vi "Create Pattern Script - Cmd Frame.vi"(8 "error in (no error)":errorcluster, 11 "BML Pattern Creater in":refnum<class "BML Pattern Creater.lvclass">) -> (0 "error out":errorcluster, 2 "CMD Frame out":string, 3 "BML Pattern Creater out":refnum<class "BML Pattern Creater.lvclass">)   [LabVIEW 2018, in "BML Pattern Creater.lvlib" / "BML Pattern Creater.lvclass"]
uses:
  BML Pattern Creater.lvclass
  Special Frame.ctl
  BML Pattern Creater.lvclass/BML Pattern Creater.ctl
  Interfaces/Protocol Interface.lvlibp/Interfaces/Protocol Interface/Pin State.ctl
  Read Frame Data.vi
  Interfaces/Protocol Interface.lvlibp/Interfaces/Protocol Interface/Protocol Interface.lvclass
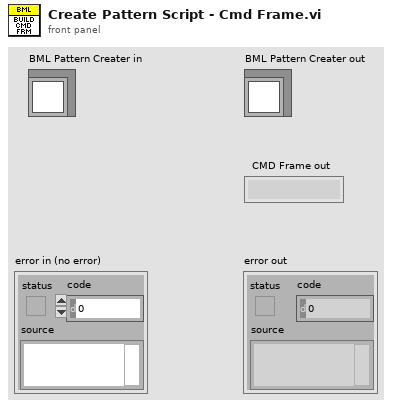
[diagram p1: front panel]
types:
  T1 = typedef "BML Pattern Creater.lvlib/BML Pattern Creater.lvclass/Special Frame.ctl" = enum16{"Sync Header", "BML Header", "SW Trig", "SetID State", "Exit SetID State", "SW Reset", "Wait"}
  T2 = typedef "FRM Data - BML.ctl" = cluster{"Pattern_Name":string, "Data":u8[], "Start_Addr":u16, "ChipID":u8, "num of wait ms":i8, "Opcode":string[], "BML OM":T3, "BurstLength":T4, "FSN":u8, "R/W?":T5}
  T3 = typedef "OM - BML.ctl" = enum16{"Normal", "ImmeEffect", "InitSlaveID", "LoadData"}
  T4 = typedef "Burst Length.ctl" = enum8{"0", "2", "3", "4", "5", "8", "16", "32"}
  T5 = typedef "RW Options.ctl" = enum16{"Read", "Write", "R/W"}
  T6 = typedef "Protocol Interface.lvlibp/Protocol Interface.lvclass/Pin State.ctl" = enum16{"0", "1", "L", "H", "X", "V", "D", "M"}
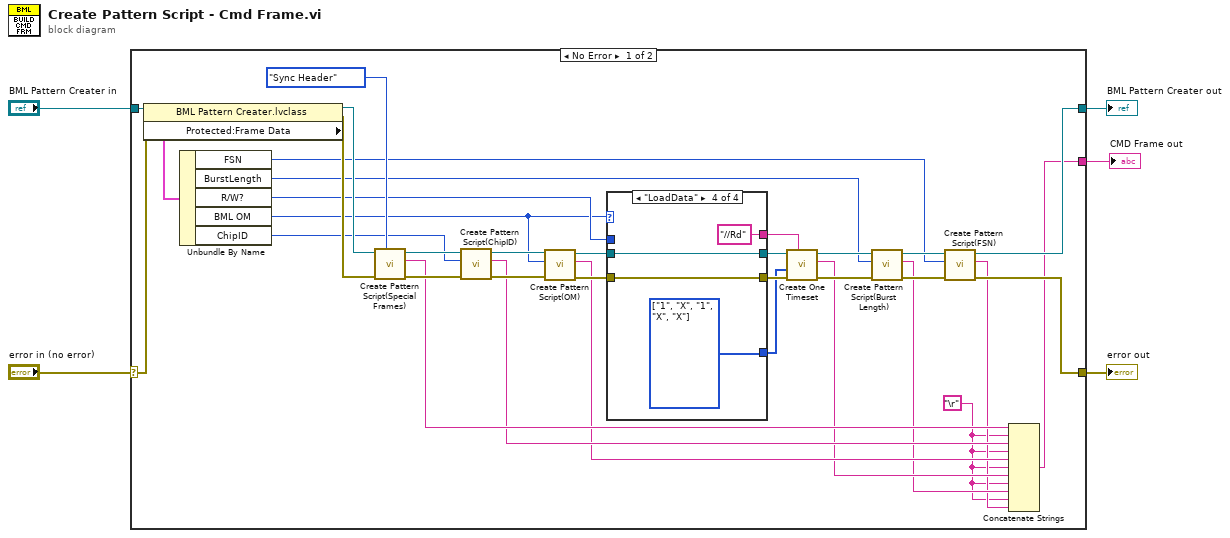
[diagram p0: block diagram]
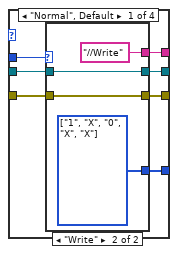
[diagram p2: hidden frame]
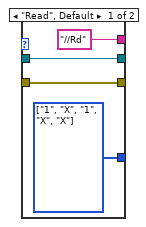
[diagram p3: hidden frame]
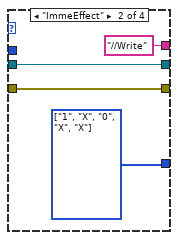
[diagram p4: hidden frame]
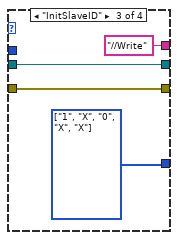
[diagram p5: hidden frame]
diagram:
  n1 = case shown="No Error" "error in (no error)" {
    selector: "error in (no error)" -> [w39 w69]
    tunnel: [w14 w69] -> w4
    tunnel: [w15 w68] -> w2
    tunnel: "BML Pattern Creater in" -> [w40 w68]
    tunnel: [w6 _] -> w1
    frame No Error {
      w7 = "\r"
      n2 = property class="BML Pattern Creater.lvclass"(reference=w40, error in=w39) -> (reference out=w37:refnum<class "BML Pattern Creater.lvclass">, error out=w36:errorcluster, "Protected:Frame Data"=w38:T2)
      n3 = Unbundle By Name(w38) -> ("FSN"=w16:u8, "BurstLength"=w17:T4, "R/W?"=w27:T5, "BML OM"=w19:T3, "ChipID"=w32:u8)
      n4 = call "Create Pattern Script(Special Frames).vi"("Special Frame Type"=Special_Frame."Sync Header", "error in (no error)"=w36, "BML Pattern Creater in"=w37) -> ("error out"=w33:errorcluster, "string out"=w13:string, "BML Pattern Creater out"=w34:refnum<class "BML Pattern Creater.lvclass">)  [unwired: 6 in]
      n5 = call "Create Pattern Script(ChipID).vi"("error in (no error)"=w33, "ChipID"=w32, "BML Pattern Creater in"=w34) -> ("error out"=w31:errorcluster, "Script out"=w12:string, "BML Pattern Creater out"=w30:refnum<class "BML Pattern Creater.lvclass">)  [unwired: 6 in]
      n6 = call "Create Pattern Script(OM).vi"("error in (no error)"=w31, "BML OM"=w19, "BML Pattern Creater in"=w30) -> ("error out"=w26:errorcluster, "OM string out"=w11:string, "BML Pattern Creater out"=w25:refnum<class "BML Pattern Creater.lvclass">)  [unwired: 6 in]
      n7 = case shown="\"LoadData\"" w19 {
        tunnel: w27 -> [w47 _ _ _]
        tunnel: w26 -> [w46 w57 w61 w65]
        tunnel: w25 -> [w45 w58 w62 w66]
        tunnel: [w44 w57 w61 w65] -> w24
        tunnel: [w43 w59 w63 w67] -> w22
        tunnel: [w42 "//Write" "//Write" "//Rd"] -> w21
        tunnel: [w41 w58 w62 w66] -> w20
        frame "Normal", Default {
          n8 = case shown="\"Write\"" w47 {
            tunnel: w46 -> [w50 w54]
            tunnel: w45 -> [w51 w55]
            tunnel: [w51 w55] -> w41
            tunnel: [w50 w54] -> w44
            tunnel: [w49 w53] -> w43
            tunnel: ["//Rd" "//Write"] -> w42
            frame "Read", Default {
              w49 = T6[] [enum."1", enum."X", enum."1", enum."X", enum."X"] items=["0", "1", "L", "H", "X", "V", "D", "M"]
            }
            frame "Write" {
              w53 = T6[] [enum."1", enum."X", enum."0", enum."X", enum."X"] items=["0", "1", "L", "H", "X", "V", "D", "M"]
            }
          }
        }
        frame "ImmeEffect" {
          w59 = T6[] [enum."1", enum."X", enum."0", enum."X", enum."X"] items=["0", "1", "L", "H", "X", "V", "D", "M"]
        }
        frame "InitSlaveID" {
          w63 = T6[] [enum."1", enum."X", enum."0", enum."X", enum."X"] items=["0", "1", "L", "H", "X", "V", "D", "M"]
        }
        frame "LoadData" {
          w67 = T6[] [enum."1", enum."X", enum."1", enum."X", enum."X"] items=["0", "1", "L", "H", "X", "V", "D", "M"]
        }
      }
      n9 = call-dynamic "Create One Timeset.vi"("Notes"=w21, "error in (no error)"=w24, "Pin State"=w22, "BML Pattern Creater in"=w20) -> ("error out"=w23:errorcluster, "string out"=w10:string, "BML Pattern Creater out"=w18:refnum<class "BML Pattern Creater.lvclass">)  [unwired: 5 in]
      n10 = call "Create Pattern Script(Burst Length).vi"("error in (no error)"=w23, "BurstLength"=w17, "BML Pattern Creater in"=w18) -> ("error out"=w29:errorcluster, "String"=w9:string, "BML Pattern Creater out"=w28:refnum<class "BML Pattern Creater.lvclass">)  [unwired: 6 in]
      n11 = call "Create Pattern Script(FSN).vi"("error in (no error)"=w29, "FSN"=w16, "BML Pattern Creater in"=w28) -> ("error out"=w14:errorcluster, "String"=w8:string, "BML Pattern Creater out"=w15:refnum<class "BML Pattern Creater.lvclass">)  [unwired: 6 in]
      n12 = Concatenate Strings(w13, w7, w12, w7, w11, w7, w10, w7, w9, w7, w8) -> (w6:string)
    }
    frame Error {
    }
  }
  "error out" <- w4
  "BML Pattern Creater out" <- w2
  "CMD Frame out" <- w1
